vi "Configure Generator ARB File Samples Subrange.vi"(6 "Stop (16)":i32=16, 7 "Start (0)":i32, 8 "error in (no error)":errorcluster, 9 "Range (Full)":i32(ring) items=["Full", "Subrange"], 10 "Instance (1)":i32=1, 11 "VISA resource name":refnum<visa-resource-name>) -> (0 "error out":errorcluster, 3 "VISA resource name out":refnum<visa-resource-name>)   [LabVIEW 2015, in "Rohde&Schwarz CMXP GPRF.lvlib"]
doc: "Defines the subrange of samples from the loaded ARB file that shall be processed by the arbitrary signal generator.\nEither the full file (all samples) or a subrange starting with the first sample can be processed.\n\nAttribute:\n-\n\nRemote-control command:\nSOURce:GPRF:GEN<i>:ARB:SAMPles:RANGe"
uses:
  <instrlib>/Rohde&Schwarz CMXP GPRF/Rohde&Schwarz CMXP GPRF.lvlib
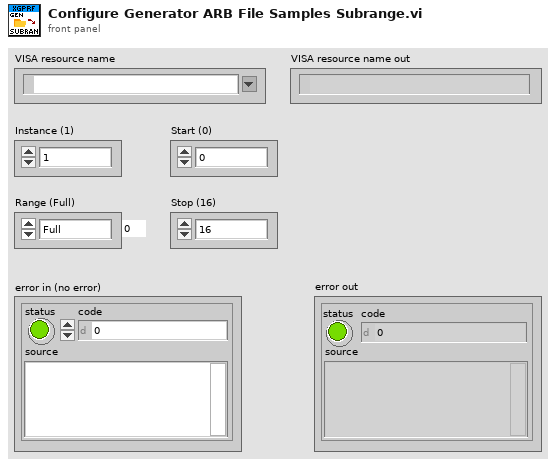
[diagram p1: front panel]
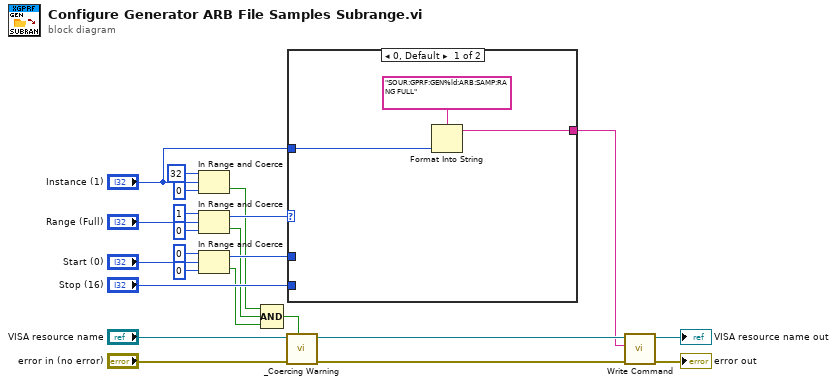
[diagram p0: block diagram]
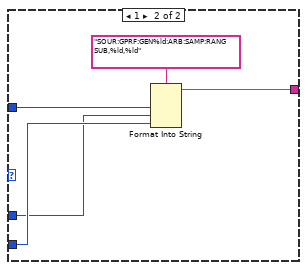
[diagram p2: hidden frame]
diagram:
  n1 = In Range and Coerce(upper limit=32, x="Instance (1)", lower limit=0) -> (In Range?=w2:bool)  [unwired: 1 out]
  n2 = In Range and Coerce(upper limit=1, x="Range (Full)", lower limit=0) -> (coerced(x)=w9:i32, In Range?=w3:bool)
  n3 = In Range and Coerce(upper limit=0, x="Start (0)", lower limit=0) -> (coerced(x)=w8:i32, In Range?=w4:bool)
  n4 = Compound Arithmetic op=AND(w2, w3, w4) -> (w17:bool)
  n5 = call <instrlib>:"_Coercing Warning.vi"("In Range?"=w17, "error in (no error)"="error in (no error)", "VISA resource name"="VISA resource name") -> ("error out"=w21:errorcluster, "VISA resource name out"=w22:refnum<visa-resource-name>)  [unwired: 7 in]
  n6 = case shown="0, Default" w9 {
    tunnel: [w26 w29] -> w1
    tunnel: "Instance (1)" -> [w24 w30]
    tunnel: w8 -> [_ w27]
    tunnel: "Stop (16)" -> [_ w28]
    frame 0, Default {
      n7 = Format Into String(format string="SOUR:GPRF:GEN%ld:ARB:SAMP:RANG FULL", w24) -> (resulting string=w26:string)  [unwired: 2 in, 1 out]
    }
    frame 1 {
      n8 = Format Into String(format string="SOUR:GPRF:GEN%ld:ARB:SAMP:RANG SUB,%ld,%ld", w30, w27, w28) -> (resulting string=w29:string)  [unwired: 2 in, 1 out]
    }
  }
  n9 = call <instrlib>:"Write Command.vi"("error in (no error)"=w21, "Command"=w1, "VISA resource name"=w22) -> ("error out"=→"error out":errorcluster, "VISA resource name out"=→"VISA resource name out":refnum<visa-resource-name>)  [unwired: 7 in]
